vi "Servo.vi"(6 "return immediately":bool, 8 "error in (no error)":errorcluster, 9 "on/off":i32(ring) items=["Off", "On"], 10 "axis name":string, 11 "controller in":refnum<k24>) -> (0 "error out":errorcluster, 3 "controller out":refnum<k24>)   [LabVIEW 2010]
uses:
  c:/aerotech/controller/5.xx.xxx/ensemble/pc/labview/2010/bin/Aerotech.Ensemble.dll
  bin/Aerotech.Ensemble.dll
  c:/aerotech/controller/5.xx.xxx/ensemble/pc/labview/2010/bin/Aerotech.Ensemble.LabVIEW.dll
  bin/Aerotech.Ensemble.LabVIEW.dll
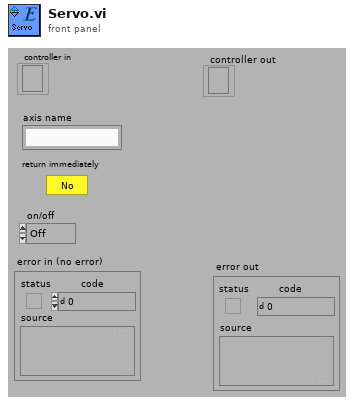
[diagram p1: front panel]
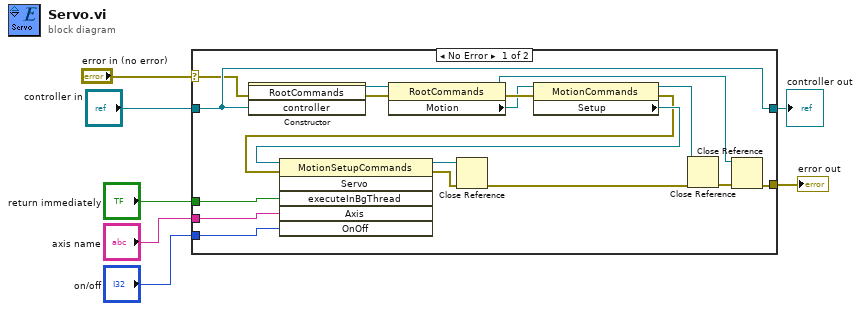
[diagram p0: block diagram]
diagram:
  n1 = case shown="No Error" "error in (no error)" {
    selector: "error in (no error)" -> [w8 w27]
    tunnel: [w14 w27] -> w6
    tunnel: "controller in" -> [w9 w26]
    tunnel: "return immediately" -> [w19 _]
    tunnel: "axis name" -> [w18 _]
    tunnel: "on/off" -> [w17 _]
    tunnel: [w9 w26] -> w1
    frame No Error {
      n2 = constructor class="RootCommands"(error in=w8, "controller"=w9) -> (reference out=w25:refnum<k24>, error out=w24:errorcluster)  [unwired: 2 in, 2 out]
      n3 = property class="RootCommands"(reference=w25, error in=w24) -> (reference out=w11:refnum<k24>, error out=w23:errorcluster, "Motion"=w22:refnum<k24>)
      n4 = property class="MotionCommands"(reference=w22, error in=w23) -> (reference out=w12:refnum<k24>, error out=w20:errorcluster, "Setup"=w21:refnum<k24>)
      n5 = invoke class="MotionSetupCommands" method="Servo"(reference=w21, error in=w20, "executeInBgThread"=w19, "Axis"=w18, "OnOff"=w17) -> (reference out=w15:refnum<k24>, error out=w16:errorcluster)  [unwired: 1 in, 4 out]
      n6 = Close Reference(reference=w15, error in (no error)=w16) -> (error out=w10:errorcluster)
      n7 = Close Reference(reference=w12, error in (no error)=w10) -> (error out=w13:errorcluster)
      n8 = Close Reference(reference=w11, error in (no error)=w13) -> (error out=w14:errorcluster)
    }
    frame Error {
    }
  }
  "error out" <- w6
  "controller out" <- w1
